vi "Updated Forward Drive Status.vi"(8 "error in (no error)":errorcluster, 11 "Forward Drive Cmd in":refnum<class "Forward Drive Cmd.lvclass">) -> (0 "error out":errorcluster, 3 "Forward Drive Cmd out":refnum<class "Forward Drive Cmd.lvclass">)   [LabVIEW 2014, in "Forward Drive.lvlib" / "Forward Drive Cmd.lvclass"]
uses:
  Forward Drive Cmd.lvclass
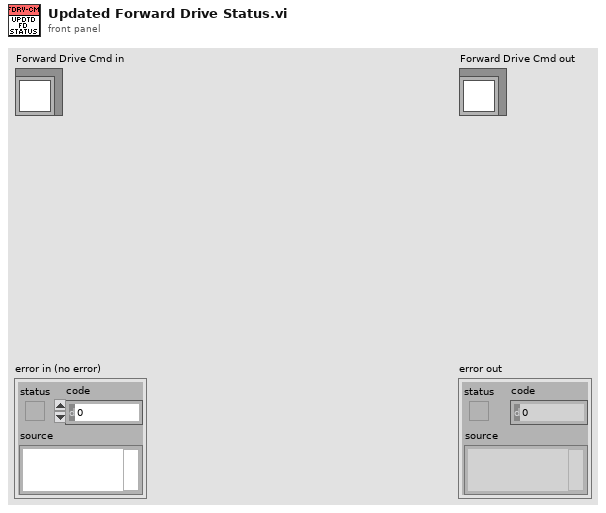
[diagram p1: front panel]
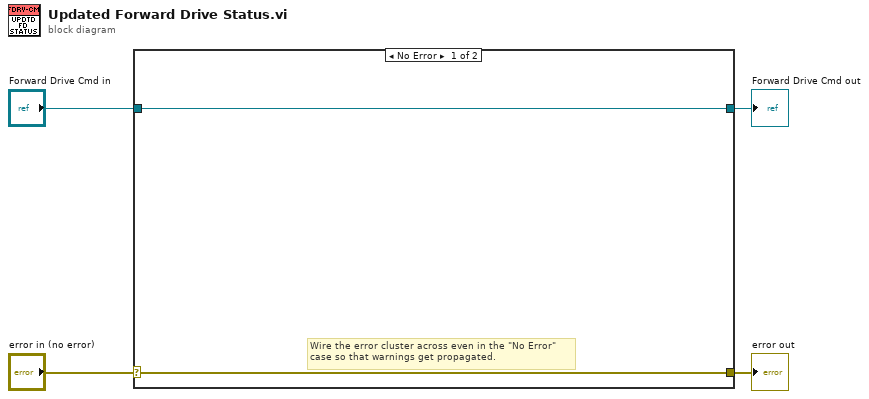
[diagram p0: block diagram]
diagram:
  n1 = case shown="No Error" "error in (no error)" {
    selector: "error in (no error)" -> [w5 w8]
    tunnel: [w5 w8] -> w3
    tunnel: [w6 w7] -> w1
    tunnel: "Forward Drive Cmd in" -> [w6 w7]
    frame No Error {
      # "Wire the error cluster across even in the \"No Error\"\ncase so that warnings get propagated."
    }
    frame Error {
    }
  }
  "error out" <- w3
  "Forward Drive Cmd out" <- w1
